vi "Init.vi"(8 "error in (no error)":errorcluster, 10 "IConfigure":refnum<class "IConfigure.lvclass">, 11 "Flir A700 in":refnum<class "Flir A700.lvclass">) -> (0 "error out":errorcluster, 3 "Flir A700 out":refnum<class "Flir A700.lvclass">)   [LabVIEW 2023, in "FLIR A700.lvlib" / "Flir A700.lvclass"]
uses:
  Flir A700.lvclass
  Interfaces/IConfigure/IConfigure.lvclass
  Camera Imaqdx/Camera Imaqdx.lvclass
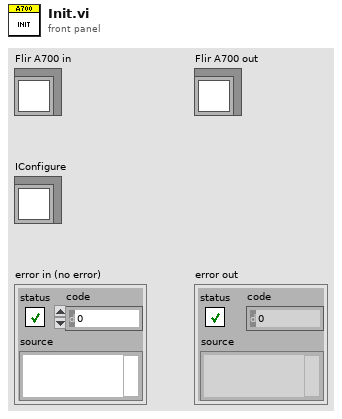
[diagram p1: front panel]
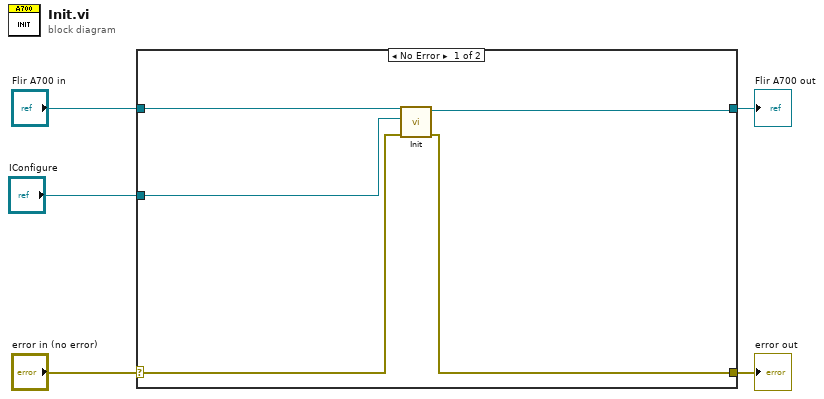
[diagram p0: block diagram]
diagram:
  n1 = case shown="No Error" "error in (no error)" {
    selector: "error in (no error)" -> [w10 w12]
    tunnel: [w8 w12] -> w4
    tunnel: [w9 w11] -> w2
    tunnel: "Flir A700 in" -> [w7 w11]
    tunnel: "IConfigure" -> [w6 _]
    frame No Error {
      n2 = call-parent "Init.vi"("error in (no error)"=w10, "IConfigure"=w6, "Camera Base in"=w7) -> ("error out"=w8:errorcluster, "Camera Base out"=w9:refnum<class "Flir A700.lvclass">)  [unwired: 7 in]
    }
    frame Error {
    }
  }
  "error out" <- w4
  "Flir A700 out" <- w2
